vi "PDF Function Trinomial Ver003.vi"(0 "NFSS Ref \nModel Value":dbl, 1 "NFSS Ref Std Dev":dbl min=0.0 step=0.1, 2 "Current Measured Value\nor Moving Window Mean":dbl, 3 "s - value":dbl) -> (14 "Probability of NEUTRAL":dbl=0.9544997361036416 format="%.6f", 16 "Prob NEGATIVE\nor DECREASING":dbl=0.02275013194817921 format="%.6f", 18 "Prob POSITIVE\nor INCREASING":dbl=0.022750131948179264 format="%.6f")   [LabVIEW 2017]
uses:
  <vilib>/gmath/NI_Gmath.lvlib
panel:
  in  "Tab Control":enum32{"Calculations", "Equations"}(tab)
  out "z - value":dbl
  out "z/sigma - s":dbl
  out "z/sigma + s":dbl
  out "Epsilon":dbl
  out "Sum of Probabilities":dbl
  # "Ref Std Dev is composed of \nthe total uncertainty due to all\ncomponents; fit, repeatability, etc.."
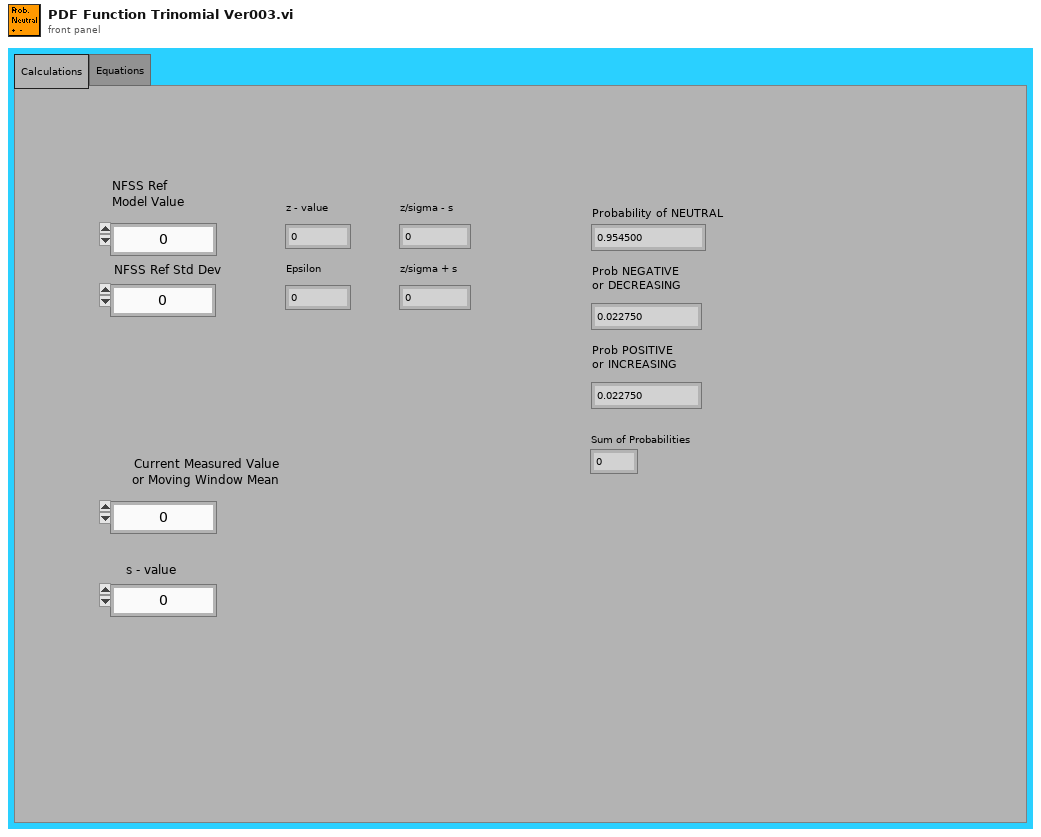
[diagram p1: front panel]
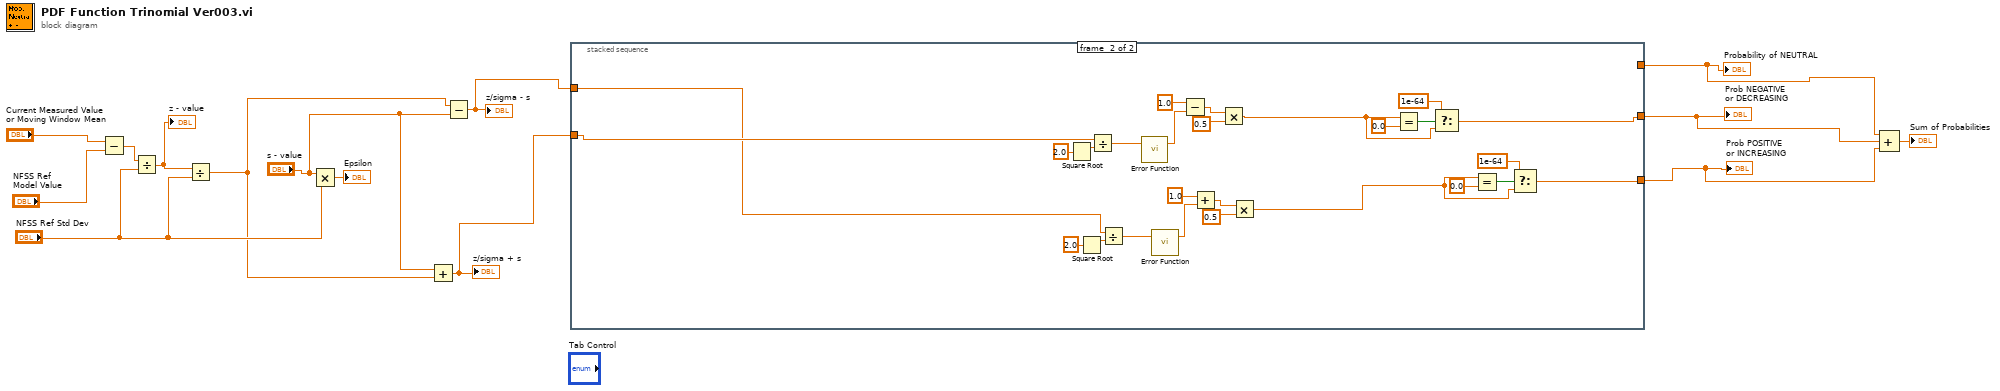
[diagram p0: block diagram]
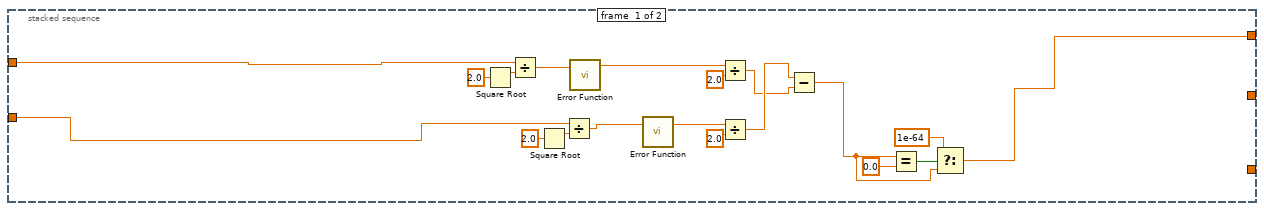
[diagram p2: hidden frame]
diagram:
  n1 = Subtract(x="Current Measured Value\nor Moving Window Mean", y="NFSS Ref \nModel Value") -> (x-y=w12:dbl)
  n2 = Divide(x=w12, y="NFSS Ref Std Dev") -> (x/y=w4:dbl)
  "z - value" <- w4
  n3 = Divide(x=w4, y="NFSS Ref Std Dev") -> (x/y=w2:dbl)
  n4 = Multiply(x="s - value", y="NFSS Ref Std Dev") -> (x*y=→"Epsilon":dbl)
  n5 = Add(x="s - value", y=w2) -> (x+y=w9:dbl)
  "z/sigma + s" <- w9
  n6 = Subtract(x=w2, y="s - value") -> (x-y=w10:dbl)
  "z/sigma - s" <- w10
  n7 = stacked-sequence {
    tunnel: w10 -> [w33 w44]
    tunnel: w9 -> [w32 w56]
    tunnel: [w15 _] -> w8
    tunnel: [_ w39] -> w7
    tunnel: [_ w34] -> w6
    frame #0 {
      n8 = Square Root(x=2.0) -> (sqrt(x)=w25:dbl)
      n9 = Divide(x=w33, y=w25) -> (x/y=w23:dbl)
      n10 = Square Root(x=2.0) -> (sqrt(x)=w22:dbl)
      n11 = Divide(x=w32, y=w22) -> (x/y=w20:dbl)
      n12 = call <vilib>:"Error Function.vi"("x"=w23) -> ("erf(x)"=w28:dbl)  [unwired: 2 out]
      n13 = call <vilib>:"Error Function.vi"("x"=w20) -> ("erf(x)"=w31:dbl)  [unwired: 2 out]
      n14 = Divide(x=w28, y=2.0) -> (x/y=w26:dbl)
      n15 = Divide(x=w31, y=2.0) -> (x/y=w27:dbl)
      n16 = Subtract(x=w27, y=w26) -> (x-y=w16:dbl)
      n17 = Equal?(x=w16, y=0.0) -> (x = y?=w19:bool)
      n18 = Select(t=1e-64 ("y"), s=w19, f=w16) -> (s? t:f=w15:dbl)
    }
    frame #1 {
      n19 = Square Root(x=2.0) -> (sqrt(x)=w59:dbl)
      n20 = Square Root(x=2.0) -> (sqrt(x)=w51:dbl)
      n21 = Divide(x=w56, y=w59) -> (x/y=w57:dbl)
      n22 = Divide(x=w44, y=w51) -> (x/y=w49:dbl)
      n23 = call <vilib>:"Error Function.vi"("x"=w57) -> ("erf(x)"=w55:dbl)  [unwired: 2 out]
      n24 = call <vilib>:"Error Function.vi"("x"=w49) -> ("erf(x)"=w48:dbl)  [unwired: 2 out]
      n25 = Subtract(x=1.0, y=w55) -> (x-y=w53:dbl)
      n26 = Add(x=1.0, y=w48) -> (x+y=w46:dbl)
      n27 = Multiply(x=w53, y=0.5) -> (x*y=w40:dbl)
      n28 = Multiply(x=w46, y=0.5) -> (x*y=w35:dbl)
      n29 = Equal?(x=w40, y=0.0) -> (x = y?=w41:bool)
      n30 = Select(t=1e-64 ("y"), s=w41, f=w40) -> (s? t:f=w39:dbl)
      n31 = Equal?(x=w35, y=0.0) -> (x = y?=w36:bool)
      n32 = Select(t=1e-64 ("y"), s=w36, f=w35) -> (s? t:f=w34:dbl)
    }
  }
  "Probability of NEUTRAL" <- w8
  "Prob NEGATIVE\nor DECREASING" <- w7
  "Prob POSITIVE\nor INCREASING" <- w6
  n33 = Compound Arithmetic op=ADD(w8, w7, w6) -> (→"Sum of Probabilities":dbl)
